vi "Reposition Wheels.vi"(5 "x positions":dbl[](array[numeric]), 6 "frame angles (rad)":dbl[](array[numeric]), 7 "y positions":dbl[](array[numeric]), 8 "error in (no error)":errorcluster, 10 "wheel indexes":i32[](array[numeric]), 11 "steering frame in":refnum<class "NI_Robotics_Steering Frame.lvclass">) -> (0 "error out":errorcluster, 1 "found?":bool[](array[boolean]), 3 "steering frame out":refnum<class "NI_Robotics_Steering Frame.lvclass">)   [LabVIEW 2017, in "NI_Robotics_Steering Frame.lvclass"]
uses:
  <vilib>/robotics/Steering/Steering Frame/NI_Robotics_Steering Frame.lvclass
  <vilib>/robotics/Steering/Steering Frame/NI_Robotics_Steering Frame.lvclass/NI_Robotics_Steering Frame.ctl
  <vilib>/robotics/Steering/Wheel/NI_Robotics_Wheel.lvclass/NI_Robotics_Wheel.ctl
  <vilib>/Analysis/coordinate.llb/Wrap Angle (scalar).vi
  <vilib>/robotics/Steering/Wheel/NI_Robotics_Wheel.lvclass
  <vilib>/Analysis/NI_AAL_Angle.lvlib
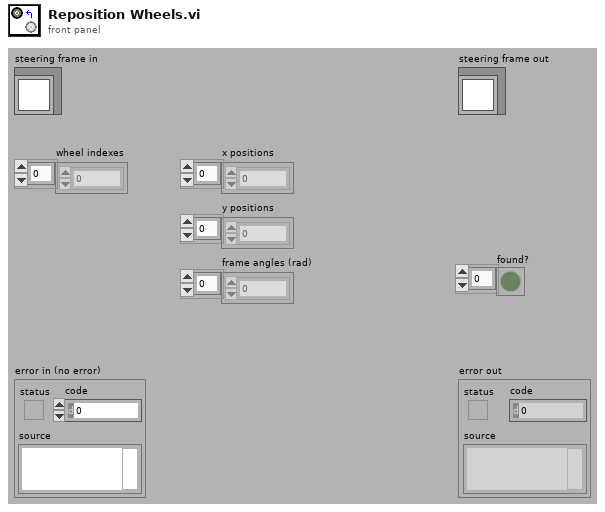
[diagram p1: front panel]
types:
  T1 = typedef "NI_Robotics_Steering Frame.lvclass/Wheel Orientation.ctl" = cluster{"wheel":refnum<class "NI_Robotics_Wheel.lvclass">, "x position":dbl, "y position":dbl, "frame angle (rad)":dbl}
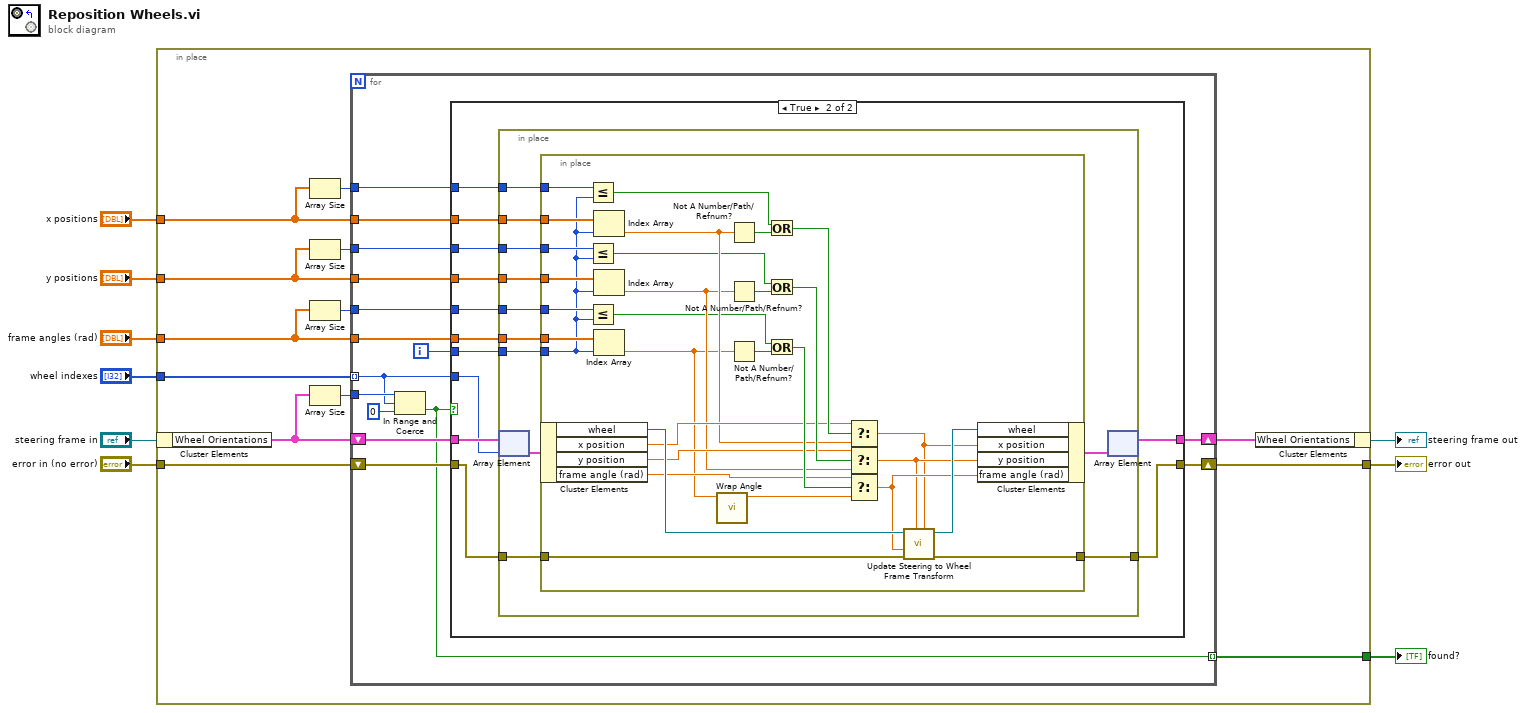
[diagram p0: block diagram]
diagram:
  n1 = in-place {
    in-place-border: "error in (no error)" -> [w18]
    in-place-border: "wheel indexes" -> [w20]
    in-place-border: [w17] -> w8
    in-place-border: [w16] -> w4
    in-place-border: "x positions" -> [w15]
    in-place-border: "y positions" -> [w14]
    in-place-border: "frame angles (rad)" -> [w13]
    n2 = in-place-cluster #1("steering frame in") -> ("Wheel Orientations"=w22:T1[])
    n3 = Array Size(array=w15) -> (size(s)=w12:i32)
    n4 = Array Size(array=w14) -> (size(s)=w11:i32)
    n5 = Array Size(array=w13) -> (size(s)=w10:i32)
    n6 = Array Size(array=w22) -> (size(s)=w19:i32)
    n7 = for {
      shift-right: [w33] -> w21
      shift-left: w22 -> [w34]
      tunnel: w20 -> [w35] mode=indexing
      tunnel: w19 -> [w36]
      shift-right: [w31] -> w17
      shift-left: w18 -> [w32]
      tunnel: [w30] -> w16 mode=indexing
      tunnel: w15 -> [w29]
      tunnel: w14 -> [w28]
      tunnel: w13 -> [w27]
      tunnel: w12 -> [w25]
      tunnel: w11 -> [w24]
      tunnel: w10 -> [w23]
      i -> [w26]
      n8 = In Range and Coerce(upper limit=w36, x=w35, lower limit=0) -> (In Range?=w30:bool)  [unwired: 1 out]
      n9 = case shown="True" w30 {
        tunnel: w35 -> [_ w50]
        tunnel: w34 -> [w39 w51]
        tunnel: [w39 w49] -> w33
        tunnel: w32 -> [w38 w46]
        tunnel: [w38 w44] -> w31
        tunnel: w29 -> [_ w48]
        tunnel: w28 -> [_ w47]
        tunnel: w27 -> [_ w45]
        tunnel: w26 -> [_ w43]
        tunnel: w25 -> [_ w42]
        tunnel: w24 -> [_ w41]
        tunnel: w23 -> [_ w40]
        frame False {
          # "Index is out of range.  Do nothing."
        }
        frame True {
          n10 = in-place {
            in-place-border: w48 -> [w59]
            in-place-border: w47 -> [w58]
            in-place-border: w46 -> [w61]
            in-place-border: w45 -> [w57]
            in-place-border: [w56] -> w44
            in-place-border: w43 -> [w55]
            in-place-border: w42 -> [w54]
            in-place-border: w41 -> [w53]
            in-place-border: w40 -> [w52]
            n11 = in-place-array #2(w51, w50) -> (w62:T1)
            n12 = in-place {
              in-place-border: w61 -> [w90]
              in-place-border: w59 -> [w76]
              in-place-border: w58 -> [w74]
              in-place-border: w57 -> [w72]
              in-place-border: [w85] -> w56
              in-place-border: w55 -> [w68]
              in-place-border: w54 -> [w71]
              in-place-border: w53 -> [w70]
              in-place-border: w52 -> [w69]
              n13 = in-place-cluster #3(w62) -> ("wheel"=w92:refnum<class "NI_Robotics_Wheel.lvclass">, "x position"=w78:dbl, "y position"=w82:dbl, "frame angle (rad)"=w87:dbl)
              n14 = Less Or Equal?(x=w71, y=w68) -> (x <= y?=w67:bool)
              n15 = Less Or Equal?(x=w70, y=w68) -> (x <= y?=w66:bool)
              n16 = Less Or Equal?(x=w69, y=w68) -> (x <= y?=w65:bool)
              n17 = Index Array(array=w76, index=w68) -> (element=w75:dbl)
              n18 = Index Array(array=w74, index=w68) -> (element=w73:dbl)
              n19 = Index Array(array=w72, index=w68) -> (element=w64:dbl)
              n20 = call-poly <vilib>:"Wrap Angle.vi"("angle in"=w64) -> ("angle out"=w63:dbl)  [unwired: 9 in, 1 out]
              n21 = Not A Number/Path/Refnum?(number/path/refnum=w75) -> (NaN/Path/Refnum?=w80:bool)
              n22 = Not A Number/Path/Refnum?(number/path/refnum=w73) -> (NaN/Path/Refnum?=w84:bool)
              n23 = Not A Number/Path/Refnum?(number/path/refnum=w64) -> (NaN/Path/Refnum?=w89:bool)
              n24 = Or(x=w67, y=w80) -> (x .or. y?=w79:bool)
              n25 = Or(x=w66, y=w84) -> (x .or. y?=w83:bool)
              n26 = Or(x=w65, y=w89) -> (x .or. y?=w88:bool)
              n27 = Select(t=w78, s=w79, f=w75) -> (s? t:f=w77:dbl)
              n28 = Select(t=w82, s=w83, f=w73) -> (s? t:f=w81:dbl)
              n29 = Select(t=w87, s=w88, f=w63) -> (s? t:f=w86:dbl)
              n30 = call <vilib>:"Update Steering to Wheel Frame Transform.vi"("x wheel position"=w77, "y wheel position"=w81, "error in (no error)"=w90, "wheel frame angle (rad)"=w86, "wheel in"=w92) -> ("error out"=w85:errorcluster, "wheel out"=w91:refnum<class "NI_Robotics_Wheel.lvclass">)  [unwired: 5 in]
              n31 = in-place-cluster #3("wheel"=w91, "x position"=w77, "y position"=w81, "frame angle (rad)"=w86) -> (w60:T1)
            }
            n32 = in-place-array #2(w60) -> (w49:T1[])  [unwired: 1 out]
          }
        }
      }
    }
    n33 = in-place-cluster #1("Wheel Orientations"=w21) -> (→"steering frame out":refnum<class "NI_Robotics_Steering Frame.lvclass">)
  }
  "error out" <- w8
  "found?" <- w4
